vi "test_SetItemInfoDependencies_SampleProject.vi"() -> (3 "Pass?":bool)   [LabVIEW 2019, in "Tests.SolutionBuilder.lvlib"]
uses:
  Tests.SolutionBuilder.lvlib
  SolutionBuilder/SolutionBuilder.lvclass
  SolutionBuilder/ProjectItem/ProjectItem.lvclass
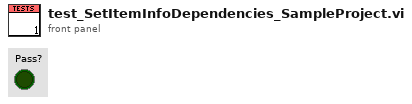
[diagram p1: front panel]
types:
  T1 = typedef "SolutionBuilder.lvlib/SolutionBuilder.lvclass/ProjectItemMap.ctl" = map{path, refnum<class "ProjectItem.lvclass">[]}
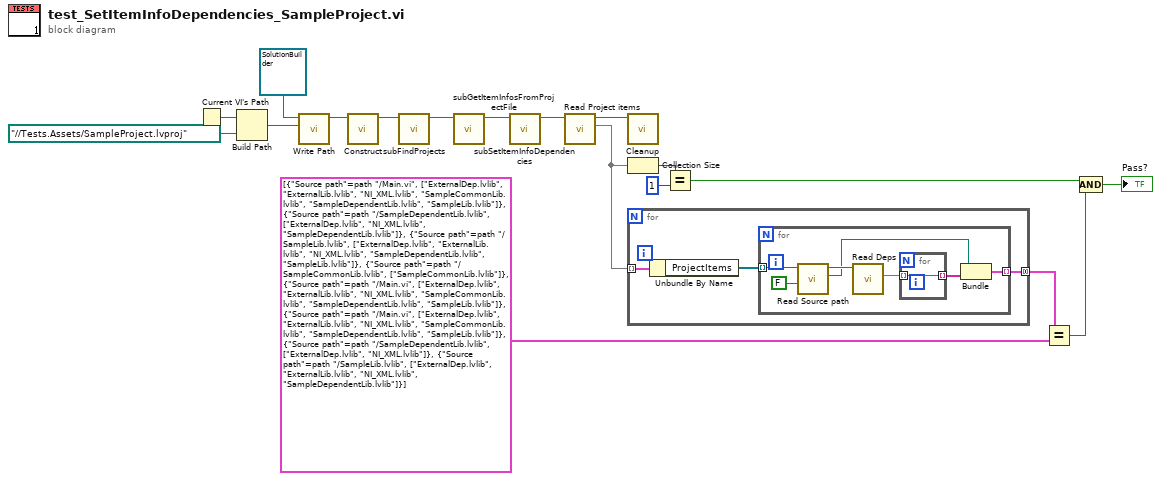
[diagram p0: block diagram]
diagram:
  n1 = Current VI's Path() -> (path=w16:path)
  n2 = Build Path(base path=w16, name or relative path=path "../../Tests.Assets/SampleProject.lvproj" ("Path")) -> (appended path=w14:path)
  n3 = call "Write Path.vi"("Path"=w14, "SolutionBuilder in"=refnum<class "SolutionBuilder.lvclass"> refnum) -> ("SolutionBuilder out"=w7:refnum<class "SolutionBuilder.lvclass">)  [unwired: 9 in]
  n4 = call "Construct.vi"("SolutionBuilder in"=w7) -> ("SolutionBuilder out"=w6:refnum<class "SolutionBuilder.lvclass">)  [unwired: 9 in, 1 out]
  n5 = call "subFindProjects.vi"("SolutionBuilder in"=w6) -> ("SolutionBuilder out"=w17:refnum<class "SolutionBuilder.lvclass">)  [unwired: 9 in, 1 out]
  n6 = call "subGetItemInfosFromProjectFile.vi"("SolutionBuilder in"=w17) -> ("SolutionBuilder out"=w9:refnum<class "SolutionBuilder.lvclass">)  [unwired: 9 in, 1 out]
  n7 = call "subSetItemInfoDependencies.vi"("SolutionBuilder in"=w9) -> ("SolutionBuilder out"=w8:refnum<class "SolutionBuilder.lvclass">)  [unwired: 9 in, 1 out]
  n8 = call "Read Project items.vi"("SolutionBuilder in"=w8) -> ("Project items"=w11:T1, "SolutionBuilder out"=w4:refnum<class "SolutionBuilder.lvclass">)  [unwired: 9 in]
  n9 = call "Cleanup.vi"("SolutionBuilder in"=w4) -> ()  [unwired: 9 in, 2 out]
  n10 = Collection Size(1:w11) -> (0:w13:i32)
  n11 = for {
    tunnel: w11 -> [w21] mode=indexing
    tunnel: [w19] -> w2 mode=concatenating
    n12 = Unbundle By Name(w21) -> ("ProjectItems"=w20:refnum<class "ProjectItem.lvclass">[])
    n13 = for {
      tunnel: w20 -> [w25] mode=indexing
      tunnel: [w26] -> w19 mode=indexing
      n14 = call "Read Source path.vi"("Force abs path? (T)"=FALSE, "ProjectItem in"=w25) -> ("Source path"=w23:path, "ProjectItem out"=w24:refnum<class "ProjectItem.lvclass">)  [unwired: 8 in]
      n15 = call "Read Deps.vi"("ProjectItem in"=w24) -> ("Deps"=w28:set{string})  [unwired: 9 in, 1 out]
      n16 = for {
        tunnel: w28 -> [w29] mode=indexing
        tunnel: [w29] -> w27 mode=indexing
      }
      n17 = Bundle("Source path"=w23, w27) -> (w26:cluster{"Source path":path, string[]})  [unwired: 1 in]
    }
  }
  n18 = Equal?(x=w13, y=1) -> (x = y?=w10:bool)
  n19 = Equal?(x=w2, y=cluster{"Source path":path, string[]}[] [{"Source path"=path "../Main.vi", ["ExternalDep.lvlib", "ExternalLib.lvlib", "NI_XML.lvlib", "SampleCommonLib.lvlib", "SampleDependentLib.lvlib", "SampleLib.lvlib"]}, {"Source path"=path "../SampleDependentLib.lvlib", ["ExternalDep.lvlib", "NI_XML.lvlib", "SampleDependentLib.lvlib"]}, {"Source path"=path "../SampleLib.lvlib", ["ExternalDep.lvlib", "ExternalLib.lvlib", "NI_XML.lvlib", "SampleDependentLib.lvlib", "SampleLib.lvlib"]}, {"Source path"=path "../SampleCommonLib.lvlib", ["SampleCommonLib.lvlib"]}, {"Source path"=path "../Main.vi", ["ExternalDep.lvlib", "ExternalLib.lvlib", "NI_XML.lvlib", "SampleCommonLib.lvlib", "SampleDependentLib.lvlib", "SampleLib.lvlib"]}, {"Source path"=path "../Main.vi", ["ExternalDep.lvlib", "ExternalLib.lvlib", "NI_XML.lvlib", "SampleCommonLib.lvlib", "SampleDependentLib.lvlib", "SampleLib.lvlib"]}, {"Source path"=path "../SampleDependentLib.lvlib", ["ExternalDep.lvlib", "NI_XML.lvlib"]}, {"Source path"=path "../SampleLib.lvlib", ["ExternalDep.lvlib", "ExternalLib.lvlib", "NI_XML.lvlib", "SampleDependentLib.lvlib"]}] ("Array")) -> (x = y?=w5:bool)
  n20 = Compound Arithmetic op=AND(w10, w5) -> (→"Pass?":bool)
